vi "S2C_Access_TableDelete.vi"(8 "Error In":errorcluster, 10 "Row":i32, 11 "Table":string) -> (0 "Error Out":errorcluster)   [LabVIEW 2015]
uses:
  S2C_Access_Globals.vi
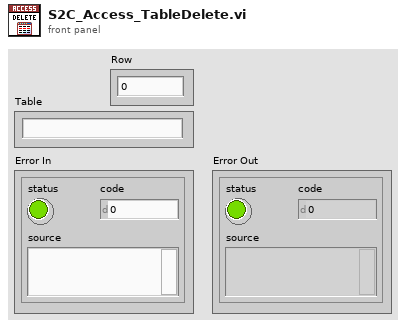
[diagram p1: front panel]
types:
  T1 = typedef "S2C_Access_Select.ctl" = string
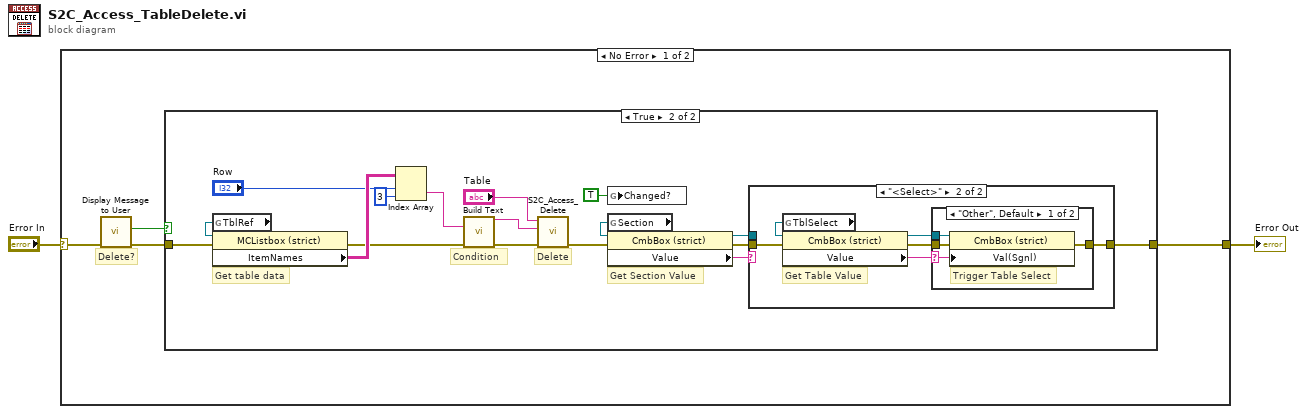
[diagram p0: block diagram]
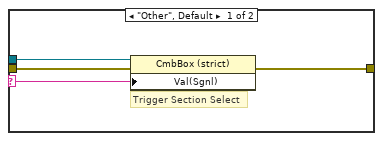
[diagram p3: hidden frame]
diagram:
  n1 = case shown="No Error" "Error In" {
    selector: "Error In" -> [w5 w40]
    tunnel: [w6 w40] -> w1
    frame No Error {
      # "Delete?"
      n2 = call "Display Message to User"("error in (no error)"=w5) -> ("error out"=w4:errorcluster, "OK"=w3:bool)  [unwired: 9 in]
      n3 = case shown="True" w3 {
        tunnel: [w7 w13] -> w6
        tunnel: w4 -> [w7 w23]
        frame False {
        }
        frame True {
          # "Get Section Value"
          # "Get table data"
          # "Delete"
          # "Condition"
          n4 = global read "S2C_Access_Globals.vi" "TblRef"() -> (w24:refnum<vi>)
          n5 = property class="MCListbox (strict)"(reference=w24, error in=w23) -> (error out=w18:errorcluster, "ItemNames"=w22:string[][])  [unwired: 1 out]
          n6 = Index Array(array=w22, index (row)="Row", index (col)=3 ("disabled index (col)")) -> (element=w17:string)
          n7 = call "Build Text"("ID"=w17, "error in (no error)"=w18) -> ("Result"=w19:string, "error out"=w20:errorcluster)  [unwired: 12 in]
          n8 = call "S2C_Access_Delete.vi"("Error In"=w20, "Condition"=w19, "Table"="Table") -> ("Error Out"=w8:errorcluster)  [unwired: 8 in]
          n9 = global write "S2C_Access_Globals.vi" "Changed?"(TRUE ("Changed?")) -> ()
          n10 = global read "S2C_Access_Globals.vi" "Section"() -> (w12:refnum<vi>)
          n11 = property class="CmbBox (strict)"(reference=w12, error in=w8) -> (reference out=w9:refnum<vi>, error out=w10:errorcluster, "Value"=w11:T1)
          n12 = case shown="\"<Select>\"" w11 {
            selector: w11 -> [w27 _]
            tunnel: w10 -> [w28 w30]
            tunnel: w9 -> [w26 _]
            tunnel: [w25 w29] -> w13
            frame "Other", Default {
              # "Trigger Section Select"
              n13 = property class="CmbBox (strict)"(reference=w26, error in=w28, "Val(Sgnl)"=w27) -> (error out=w25:errorcluster)  [unwired: 1 out]
            }
            frame "<Select>" {
              # "Get Table Value"
              n14 = global read "S2C_Access_Globals.vi" "TblSelect"() -> (w34:refnum<vi>)
              n15 = property class="CmbBox (strict)"(reference=w34, error in=w30) -> (reference out=w31:refnum<vi>, error out=w33:errorcluster, "Value"=w32:T1)
              n16 = case shown="\"Other\", Default" w32 {
                selector: w32 -> [w35 _]
                tunnel: w33 -> [w38 w39]
                tunnel: w31 -> [w37 _]
                tunnel: [w36 w39] -> w29
                frame "Other", Default {
                  # "Trigger Table Select"
                  n17 = property class="CmbBox (strict)"(reference=w37, error in=w38, "Val(Sgnl)"=w35) -> (error out=w36:errorcluster)  [unwired: 1 out]
                }
                frame "<Select>" {
                  # "Table not selected"
                }
              }
            }
          }
        }
      }
    }
    frame Error {
    }
  }
  "Error Out" <- w1
